vi "Reset.vi"(8 "error in (no error)":errorcluster, 11 "VISA resource name":refnum<visa-resource-name>) -> (0 "error out":errorcluster, 3 "VISA resource name out":refnum<visa-resource-name>)   [LabVIEW 2017, in "GP22_TDC_Arduinoed.lvlib"]
doc: "Resets the instrument and then sends a set of default setup commands to the instrument."
uses:
  GP22_TDC_Arduinoed.lvlib
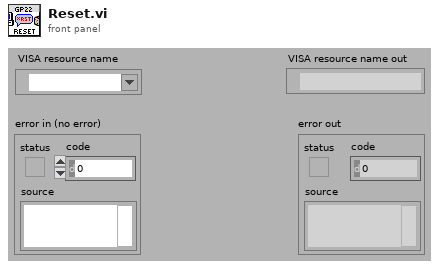
[diagram p1: front panel]
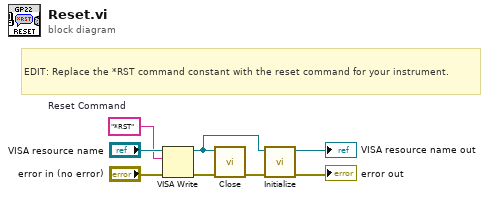
[diagram p0: block diagram]
diagram:
  w5 = "*RST"  # Reset Command
  # "EDIT: Replace the *RST command constant with the reset command for your instrument."
  n1 = VISA Write(VISA resource name="VISA resource name", write buffer=w5, error in (no error)="error in (no error)") -> (VISA resource name out=w1:refnum<visa-resource-name>, error out=w4:errorcluster)  [unwired: 1 out]
  n2 = call "Close.vi"("VISA resource name"=w1) -> ()  [unwired: 10 in, 1 out]
  n3 = call "Initialize.vi"("error in (no error)"=w4, "VISA resource name"=w1) -> ("error out"=→"error out":errorcluster, "VISA resource name out"=→"VISA resource name out":refnum<visa-resource-name>)  [unwired: 8 in]
